vi "Generate Alarms Log File Header.vi"() -> (3 "Header":string)   [LabVIEW 2015, in "Alarm Handler Actor.lvclass"]
uses:
  Alarm Handler Actor.lvclass
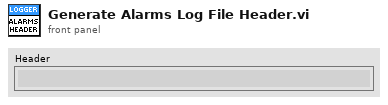
[diagram p1: front panel]
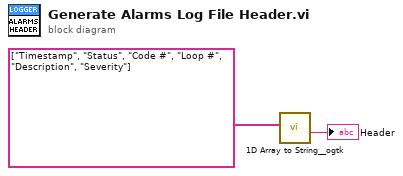
[diagram p0: block diagram]
diagram:
  n1 = call <userlib>:"1D Array to String__ogtk.vi"("Array of Strings"=string[] ["Timestamp", "Status", "Code #", "Loop #", "Description", "Severity"]) -> ("delimited string"=→"Header":string)  [unwired: 10 in]
